vi "Scan properties and methods.vi"() -> ()   [LabVIEW 2019, in "Scan Engine Custom Device.lvlib"]
uses:
  Scan Engine Custom Device.lvlib
  <resource>/objmgr/ni.var.rc
  <resource>/objmgr/IndComECAT.rc
  <resource>/objmgr/cRIO.rc
panel:
  out "Slot":u32
  out "Model":u32
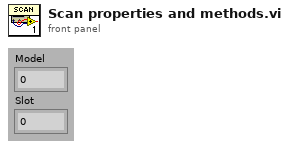
[diagram p1: front panel]
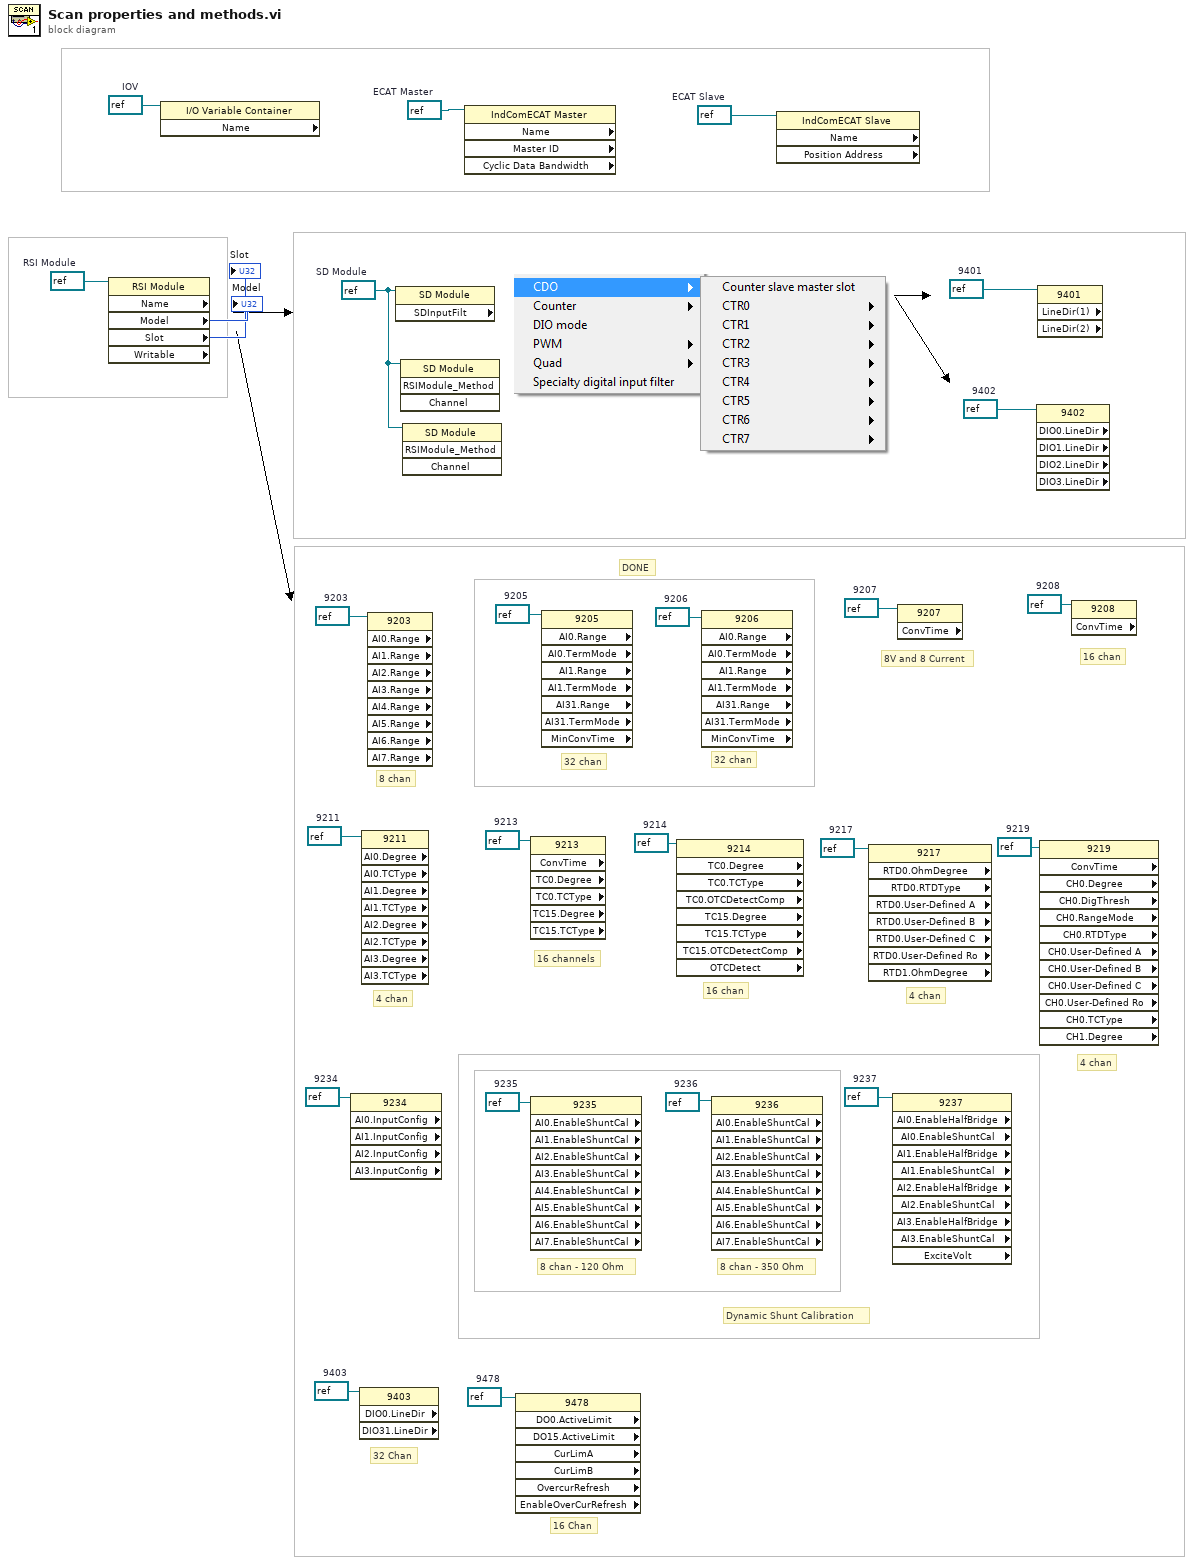
[diagram p0: block diagram]
diagram:
  w3 = refnum<k21> refnum  # 9478
  w4 = refnum<k21> refnum  # 9403
  w5 = refnum<k21> refnum  # 9237
  w6 = refnum<k21> refnum  # 9236
  w7 = refnum<k21> refnum  # 9235
  w8 = refnum<k21> refnum  # 9234
  w9 = refnum<k21> refnum  # 9219
  w10 = refnum<k21> refnum  # 9217
  w13 = refnum<k21> refnum  # 9214
  w14 = refnum<k21> refnum  # 9213
  w15 = refnum<k21> refnum  # 9211
  w16 = refnum<k21> refnum  # 9208
  w17 = refnum<k21> refnum  # 9207
  w18 = refnum<k21> refnum  # 9206
  w19 = refnum<k21> refnum  # 9205
  w20 = refnum<k21> refnum  # 9203
  w11 = refnum<k21> refnum  # 9402
  w12 = refnum<k21> refnum  # 9401
  w21 = refnum<k21> refnum  # SD Module
  w22 = refnum<k21> refnum  # RSI Module
  w23 = refnum<k21> refnum  # ECAT Slave
  w24 = refnum<k21> refnum  # ECAT Master
  w25 = refnum<k21> refnum  # IOV
  # "DONE"
  # "16 Chan"
  # "32 Chan"
  # "Dynamic Shunt Calibration"
  # "8 chan - 350 Ohm"
  # "8 chan - 120 Ohm"
  # "4 chan"
  # "4 chan"
  # "4 chan"
  # "16 chan"
  # "16 channels"
  # "16 chan"
  # "8V and 8 Current"
  # "32 chan"
  # "8 chan"
  # "32 chan"
  n1 = property class="RSI Module" props=["Name", "Model", "Slot", "Writable"](reference=w22) -> ("Model"=→"Model":u32, "Slot"=→"Slot":u32)  [unwired: 1 in, 4 out]
  n2 = property class="I/O Variable Container" props=["Name"](reference=w25) -> ()  [unwired: 1 in, 3 out]
  n3 = property class="9234" props=["AI0.InputConfig", "AI1.InputConfig", "AI2.InputConfig", "AI3.InputConfig"](reference=w8) -> ()  [unwired: 1 in, 6 out]
  n4 = property class="9403" props=["DIO0.LineDir", "DIO31.LineDir"](reference=w4) -> ()  [unwired: 1 in, 4 out]
  n5 = property class="9211" props=["AI0.Degree", "AI0.TCType", "AI1.Degree", "AI1.TCType", "AI2.Degree", "AI2.TCType", "AI3.Degree", "AI3.TCType"](reference=w15) -> ()  [unwired: 1 in, 10 out]
  n6 = property class="9203" props=["AI0.Range", "AI1.Range", "AI2.Range", "AI3.Range", "AI4.Range", "AI5.Range", "AI6.Range", "AI7.Range"](reference=w20) -> ()  [unwired: 1 in, 10 out]
  n7 = property class="SD Module" props=["SDInputFilt"](reference=w21) -> ()  [unwired: 1 in, 3 out]
  n8 = invoke class="SD Module" method="RSIModule_Method"(reference=w21) -> ()  [unwired: 3 in, 4 out]
  n9 = invoke class="SD Module" method="RSIModule_Method"(reference=w21) -> ()  [unwired: 3 in, 4 out]
  n10 = property class="IndComECAT Master" props=["Name", "Master ID", "Cyclic Data Bandwidth"](reference=w24) -> ()  [unwired: 1 in, 5 out]
  n11 = property class="9478" props=["DO0.ActiveLimit", "DO15.ActiveLimit", "CurLimA", "CurLimB", "OvercurRefresh", "EnableOverCurRefresh"](reference=w3) -> ()  [unwired: 1 in, 8 out]
  n12 = property class="9213" props=["ConvTime", "TC0.Degree", "TC0.TCType", "TC15.Degree", "TC15.TCType"](reference=w14) -> ()  [unwired: 1 in, 7 out]
  n13 = property class="9235" props=["AI0.EnableShuntCal", "AI1.EnableShuntCal", "AI2.EnableShuntCal", "AI3.EnableShuntCal", "AI4.EnableShuntCal", "AI5.EnableShuntCal", "AI6.EnableShuntCal", "AI7.EnableShuntCal"](reference=w7) -> ()  [unwired: 1 in, 10 out]
  n14 = property class="9205" props=["AI0.Range", "AI0.TermMode", "AI1.Range", "AI1.TermMode", "AI31.Range", "AI31.TermMode", "MinConvTime"](reference=w19) -> ()  [unwired: 1 in, 9 out]
  n15 = property class="9214" props=["TC0.Degree", "TC0.TCType", "TC0.OTCDetectComp", "TC15.Degree", "TC15.TCType", "TC15.OTCDetectComp", "OTCDetect"](reference=w13) -> ()  [unwired: 1 in, 9 out]
  n16 = property class="9206" props=["AI0.Range", "AI0.TermMode", "AI1.Range", "AI1.TermMode", "AI31.Range", "AI31.TermMode", "MinConvTime"](reference=w18) -> ()  [unwired: 1 in, 9 out]
  n17 = property class="9236" props=["AI0.EnableShuntCal", "AI1.EnableShuntCal", "AI2.EnableShuntCal", "AI3.EnableShuntCal", "AI4.EnableShuntCal", "AI5.EnableShuntCal", "AI6.EnableShuntCal", "AI7.EnableShuntCal"](reference=w6) -> ()  [unwired: 1 in, 10 out]
  n18 = property class="IndComECAT Slave" props=["Name", "Position Address"](reference=w23) -> ()  [unwired: 1 in, 4 out]
  n19 = property class="9217" props=["RTD0.OhmDegree", "RTD0.RTDType", "RTD0.User-Defined A", "RTD0.User-Defined B", "RTD0.User-Defined C", "RTD0.User-Defined Ro", "RTD1.OhmDegree"](reference=w10) -> ()  [unwired: 1 in, 9 out]
  n20 = property class="9237" props=["AI0.EnableHalfBridge", "AI0.EnableShuntCal", "AI1.EnableHalfBridge", "AI1.EnableShuntCal", "AI2.EnableHalfBridge", "AI2.EnableShuntCal", "AI3.EnableHalfBridge", "AI3.EnableShuntCal", "ExciteVolt"](reference=w5) -> ()  [unwired: 1 in, 11 out]
  n21 = property class="9207" props=["ConvTime"](reference=w17) -> ()  [unwired: 1 in, 3 out]
  n22 = property class="9402" props=["DIO0.LineDir", "DIO1.LineDir", "DIO2.LineDir", "DIO3.LineDir"](reference=w11) -> ()  [unwired: 1 in, 6 out]
  n23 = property class="9401" props=["LineDir(1)", "LineDir(2)"](reference=w12) -> ()  [unwired: 1 in, 4 out]
  n24 = property class="9219" props=["ConvTime", "CH0.Degree", "CH0.DigThresh", "CH0.RangeMode", "CH0.RTDType", "CH0.User-Defined A", "CH0.User-Defined B", "CH0.User-Defined C", "CH0.User-Defined Ro", "CH0.TCType", "CH1.Degree"](reference=w9) -> ()  [unwired: 1 in, 13 out]
  n25 = property class="9208" props=["ConvTime"](reference=w16) -> ()  [unwired: 1 in, 3 out]
